vi "Logger Close.vi"(11 "error in (no error)":errorcluster) -> (15 "error out":errorcluster)   [LabVIEW 2018]
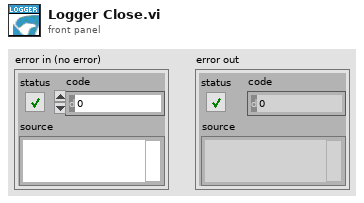
[diagram p1: front panel]
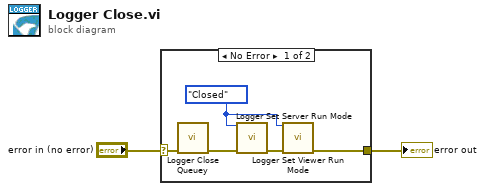
[diagram p0: block diagram]
diagram:
  n1 = case shown="No Error" "error in (no error)" {
    selector: "error in (no error)" -> [w5 w8]
    tunnel: [w4 w8] -> w1
    frame No Error {
      w3 = enum16{"Running", "Closed"}."Closed" ("Server Status")
      n2 = call "Logger Close Queuey.vi"("error in (no error)"=w5) -> ("error out"=w6:errorcluster)  [unwired: 14 in]
      n3 = call "Logger Set Server Run Mode.vi"("Server Status"=w3, "error in (no error)"=w6) -> ("error out"=w7:errorcluster)  [unwired: 13 in]
      n4 = call "Logger Set Viewer Run Mode.vi"("Server Status"=w3, "error in (no error)"=w7) -> ("error out"=w4:errorcluster)  [unwired: 13 in]
    }
    frame Error {
    }
  }
  "error out" <- w1
